vi "Modbus_Scan_Debugger.vi"(4 "reference 5":refnum<vi>, 5 "Scan debugger":bool, 6 "error in (no error)":errorcluster, 7 "reference":refnum<vi>, 8 "reference 4":refnum<vi>, 9 "reference 3":refnum<vi>, 10 "reference 2":refnum<vi>, 11 "MB_Master in":refnum<class "MB_Master.lvclass">) -> (0 "error out":errorcluster, 3 "MB_Master out":refnum<class "MB_Master.lvclass">)   [LabVIEW 2023, in "Jiaxin_Stepper_Controller.lvlib" / "Jiaxin_Stepper.lvclass"]
uses:
  Jiaxin_Stepper/Jiaxin_Stepper.lvclass
  <vilib>/Plasmionique/MB Master/MB_Master/MB_Master.lvclass
  <vilib>/Plasmionique/MB Master/MB_ADU/MB_ADU.lvclass/MB_ADU.ctl
  <vilib>/Plasmionique/MB Master/MB_ADU/Read TX Data.vi
  <vilib>/Plasmionique/MB Master/MB_ADU/Read RX Data.vi
  <vilib>/Plasmionique/MB Master/MB_ADU/Read RX Timestamp.vi
  <vilib>/Plasmionique/MB Master/MB_ADU/MB_ADU.lvclass
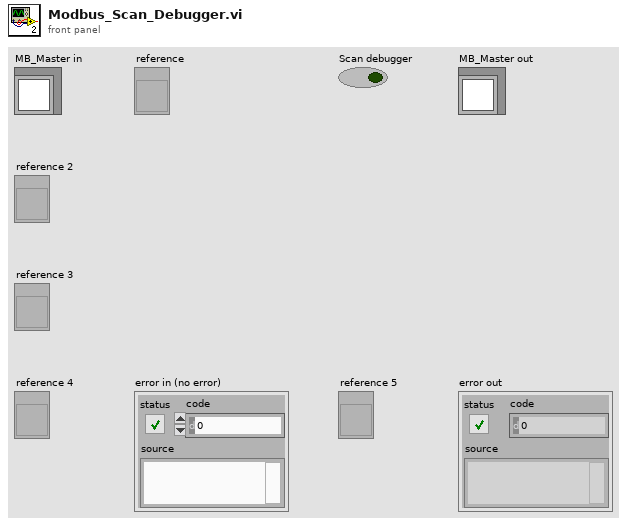
[diagram p1: front panel]
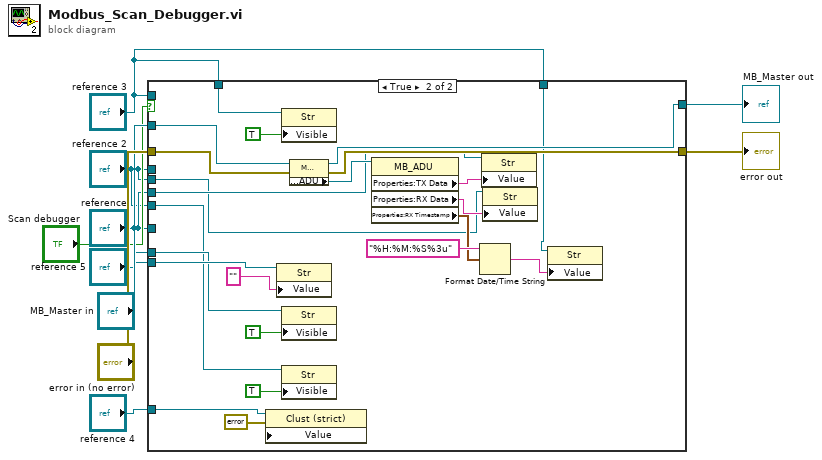
[diagram p0: block diagram]
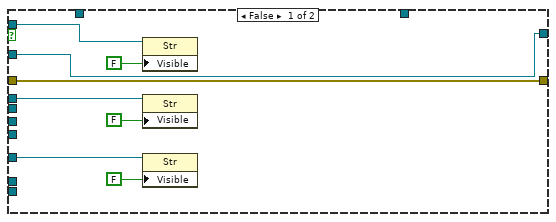
[diagram p2: hidden frame]
diagram:
  n1 = case shown="True" "Scan debugger" {
    tunnel: "MB_Master in" -> [w18 w35]
    tunnel: [w18 w39] -> w6
    tunnel: "error in (no error)" -> [w17 w34]
    tunnel: [w17 w33] -> w7
    tunnel: "reference" -> [w13 _]
    tunnel: "reference 2" -> [w12 _]
    tunnel: "reference 3" -> [w11 _]
    tunnel: "reference 4" -> [_ w26]
    tunnel: "reference 5" -> [_ w25]
    tunnel: "reference" -> [_ w24]
    tunnel: "reference 2" -> [_ w23]
    tunnel: "reference 3" -> [_ w22]
    tunnel: "reference 3" -> [_ w21]
    tunnel: "reference" -> [_ w20]
    tunnel: "reference 2" -> [_ w19]
    frame False {
      n2 = property on="Property Node" class="Str"(reference=w11, "Visible"=FALSE) -> ()  [unwired: 1 in, 2 out]
      n3 = property on="Property Node" class="Str"(reference=w12, "Visible"=FALSE) -> ()  [unwired: 1 in, 2 out]
      n4 = property on="Property Node" class="Str"(reference=w13, "Visible"=FALSE) -> ()  [unwired: 1 in, 2 out]
    }
    frame True {
      n5 = property class="Clust (strict)"(reference=w26, "Value"=errorcluster {"status"=FALSE, "code"=0, "source"=""} ("Last Error Status")) -> ()  [unwired: 1 in, 2 out]
      n6 = property class="Str"(reference=w25, "Value"="" ("Last Error Time")) -> ()  [unwired: 1 in, 2 out]
      n7 = property on="Property Node" class="Str"(reference=w22, "Visible"=TRUE) -> ()  [unwired: 1 in, 2 out]
      n8 = property on="Property Node" class="Str"(reference=w24, "Visible"=TRUE) -> ()  [unwired: 1 in, 2 out]
      n9 = property on="Property Node" class="Str"(reference=w23, "Visible"=TRUE) -> ()  [unwired: 1 in, 2 out]
      n10 = property class="MB_Master"(reference=w35, error in=w34) -> (reference out=w39:refnum<class "MB_Master.lvclass">, error out=w33:errorcluster, "Properties:ADU"=w40:refnum<class "MB_ADU.lvclass">)
      n11 = property class="MB_ADU"(reference=w40) -> ("Properties:TX Data"=w29:string, "Properties:RX Data"=w27:string, "Properties:RX Timestamp"=w36:timestamp)  [unwired: 1 in, 2 out]
      n12 = Format Date/Time String(time format string (%c)="%H:%M:%S%3u", seconds (now)=w36) -> (date/time string=w28:string)  [unwired: 1 in]
      n13 = property class="Str"(reference=w20, "Value"=w29) -> ()  [unwired: 1 in, 2 out]
      n14 = property class="Str"(reference=w19, "Value"=w27) -> ()  [unwired: 1 in, 2 out]
      n15 = property class="Str"(reference=w21, "Value"=w28) -> ()  [unwired: 1 in, 2 out]
    }
  }
  "error out" <- w7
  "MB_Master out" <- w6
